vi "GripSmart.vi"(8 "error in":errorcluster, 10 "Turn to (in)":bool, 11 "Servo":T1) -> (0 "error out":errorcluster, 3 "Turn to (out)":bool)   [LabVIEW 2017]
doc: "Servo gripper VI. \nThree grippers allowed (Left, Front,Right).\nPositions: opened and closed.\n\n1) Configure PWM frequency, conversion from degrees to duty cycle\n2) Assign PWM B channels to servo/gripper\n3) (Smart) Open PWM B channel\n4) Move servo/gripper, to open or close\n\nReturns the final position, so that state might be maintained. \n\nExecution type: Preallocated clone reentrant execution\nThe addition of the case structure is necessary to keep the correct status (channel). Otherwise the status of the VI does not correlate to the corresponding servo. Each servo (hardware) demands its own VI (software)."
uses:
  ServoEnumControl.ctl
  <vilib>/Utility/error.llb/Error Cluster From Error Code.vi
  <vilib>/myRIO/Common/Instrument Driver Framework/myRIO v1.0/PWM/vis/myRIO v1.0 Write PWM.vi
  <vilib>/myRIO/Instrument Drivers/Onboard IO/PWM/PWM.lvlib
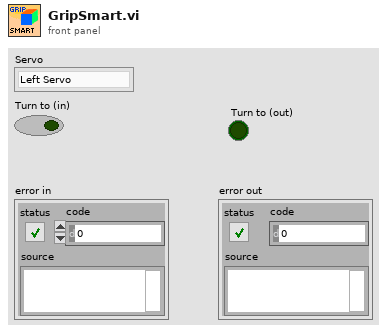
[diagram p1: front panel]
types:
  T1 = typedef "ServoEnumControl.ctl" = enum16{"Left Servo", "Front Servo", "Right Servo"}
  T2 = typedef "PWM.lvlib/PWM Reference.ctl" = cluster{"myRIO Reference":T3, "PWM Channels Enum":T7, "PWM Configuration":T8}
  T3 = typedef "myRIO Generic Hardware Reference.ctl" = cluster{"myRIO Model":T4, "myRIO Hardware Reference":T5}
  T4 = typedef "Hardware Version Enum.ctl" = enum16{"Unknown", "myRIO-1900", "myRIO-1950", "roboRIO", "NI ELVIS RIO CM"}
  T5 = typedef "myRIO v1.0 Reference.ctl" = cluster{"Generic FPGA Reference":T6, "Allow multiple opens":bool}
  T6 = typedef "Generic FPGA Reference.ctl" = refnum<k20>
  T7 = typedef "PWM Channels Enum.ctl" = enum16{"Not Connected", "C/PWM0", "C/PWM1", "A/PWM0", "A/PWM1", "A/PWM2", "B/PWM0", "B/PWM1", "B/PWM2", "PWM/PWM0", "PWM/PWM1", "PWM/PWM2", "PWM/PWM3", "PWM/PWM4", "PWM/PWM5", "PWM/PWM6", "PWM/PWM7", "PWM/PWM8", "PWM/PWM9"}
  T8 = typedef "PWM.lvlib/PWM Configuration.ctl" = cluster{"Frequency":dbl, "Duty Cycle":dbl}
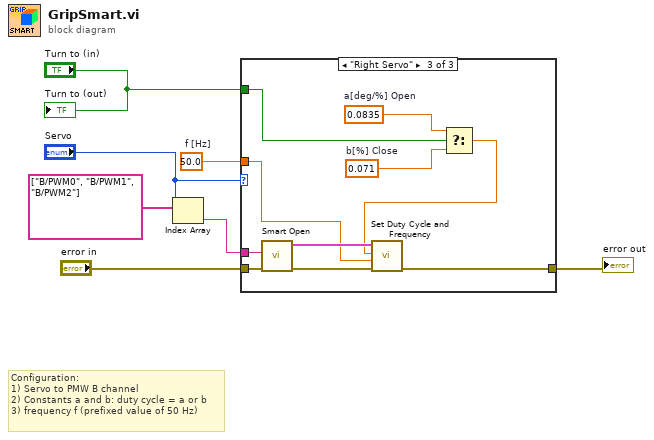
[diagram p0: block diagram]
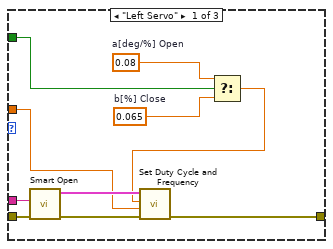
[diagram p2: hidden frame]
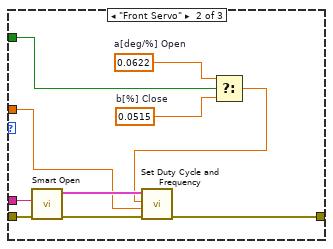
[diagram p3: hidden frame]
diagram:
  w3 = 50.0  # f [Hz]
  # "Configuration:\n1) Servo to PMW B channel\n2) Constants a and b: duty cycle = a or b\n3) frequency f (prefixed value of 50 Hz)"
  n1 = Index Array(array=tag[] ["B/PWM0", "B/PWM1", "B/PWM2"], index="Servo") -> (element=w4:tag)
  n2 = case shown="\"Right Servo\"" "Servo" {
    tunnel: "error in" -> [w10 w27 w30]
    tunnel: [w12 w24 w32] -> w6
    tunnel: w4 -> [w9 w23 w29]
    tunnel: w3 -> [w11 w22 w31]
    tunnel: "Turn to (in)" -> [w8 w19 w28]
    frame "Left Servo" {
      w14 = 0.08  # a[deg/%] Open
      w15 = 0.065  # b[%] Close
      n3 = call <vilib>:"Smart Open.vi"("error in (no error)"=w10, "Channel Name"=w9) -> ("error out"=w16:errorcluster, "PWM Ref Out"=w17:T2)  [unwired: 8 in]
      n4 = Select(t=w14, s=w8, f=w15) -> (s? t:f=w13:dbl)
      n5 = call <vilib>:"Set Duty Cycle and Frequency.vi"("error in (no error)"=w16, "Frequency [Hz]"=w11, "Duty Cycle"=w13, "PWM Ref In"=w17) -> ("error out"=w12:errorcluster)  [unwired: 5 in, 1 out]
    }
    frame "Front Servo" {
      w20 = 0.0622  # a[deg/%] Open
      w21 = 0.0515  # b[%] Close
      n6 = call <vilib>:"Smart Open.vi"("error in (no error)"=w27, "Channel Name"=w23) -> ("error out"=w25:errorcluster, "PWM Ref Out"=w26:T2)  [unwired: 8 in]
      n7 = Select(t=w20, s=w19, f=w21) -> (s? t:f=w18:dbl)
      n8 = call <vilib>:"Set Duty Cycle and Frequency.vi"("error in (no error)"=w25, "Frequency [Hz]"=w22, "Duty Cycle"=w18, "PWM Ref In"=w26) -> ("error out"=w24:errorcluster)  [unwired: 5 in, 1 out]
    }
    frame "Right Servo" {
      w34 = 0.0835  # a[deg/%] Open
      w35 = 0.071  # b[%] Close
      n9 = call <vilib>:"Smart Open.vi"("error in (no error)"=w30, "Channel Name"=w29) -> ("error out"=w36:errorcluster, "PWM Ref Out"=w37:T2)  [unwired: 8 in]
      n10 = Select(t=w34, s=w28, f=w35) -> (s? t:f=w33:dbl)
      n11 = call <vilib>:"Set Duty Cycle and Frequency.vi"("error in (no error)"=w36, "Frequency [Hz]"=w31, "Duty Cycle"=w33, "PWM Ref In"=w37) -> ("error out"=w32:errorcluster)  [unwired: 5 in, 1 out]
    }
  }
  "error out" <- w6
  "Turn to (out)" <- "Turn to (in)"
